vi "ExSubInitCam.vi"(2 "error in (no error)":errorcluster, 3 "Camera Information":T1={"acquire focus mode"=1, "Exposure"=0.0, "Number of Images"=1, "Software accumulation"=1} {"Software accumulation" min=1; "Number of Images" min=1; "Exposure" format="%.6f"; "acquire focus mode" min=1 max=4 step=1}, 4 "Camera Handle":u32) -> (0 "error out":errorcluster, 1 "Camera Handle":u32)   [LabVIEW 2010]
panel:
  # "This is a SubVI that sets the experiment mode and \ninitializes the camera."
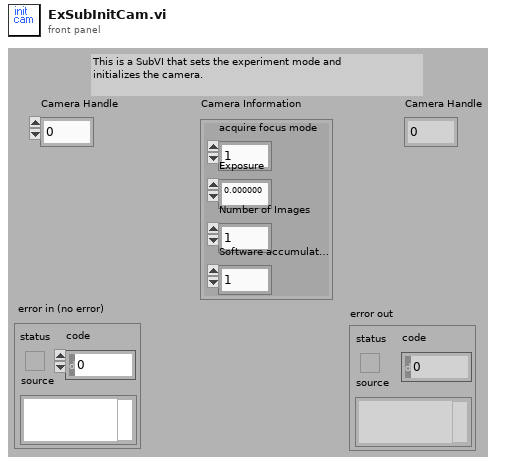
[diagram p1: front panel]
types:
  T1 = cluster{"acquire focus mode":u32, "Exposure":dbl, "Number of Images":u32, "Software accumulation":u32}
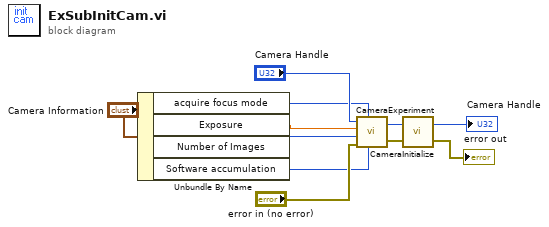
[diagram p0: block diagram]
diagram:
  n1 = Unbundle By Name("Camera Information") -> ("acquire focus mode"=w4:u32, "Exposure"=w3:dbl, "Number of Images"=w2:u32, "Software accumulation"=w1:u32)
  n2 = call <userlib>:"CameraExperiment.vi"("Number of Accumulations"=w1, "Acquire / Focus Flag"=w4, "error in"="error in (no error)", "Number of Images"=w2, "Exposure (sec)"=w3, "Camera Handle"="Camera Handle") -> ("error out"=w5:errorcluster, "Camera Handle"=w6:u32)
  n3 = call <userlib>:"CameraInitialize.vi"("error in"=w5, "Camera Handle"=w6) -> ("error out"=→"error out":errorcluster, "Camera Handle"=→"Camera Handle":u32)
